vi "PCSMain.set i Attri.vi"(2 "error in (no error)":errorcluster, 3 "systemID":string) -> (0 "error out":errorcluster, 1 "i attribute":T1)   [LabVIEW 2014, in "PCSMain.lvlib"]
uses:
  PCSMain.lvlib
  PCSMain.i attribute.ctl
  PH_Common/PH_Common.lvlib
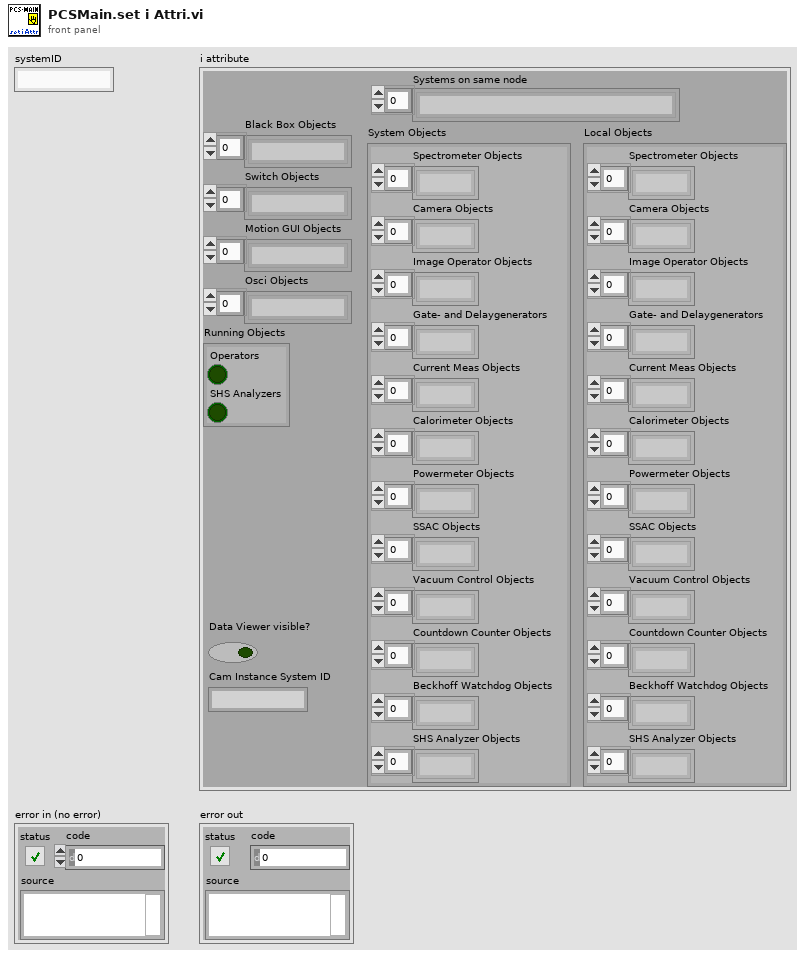
[diagram p1: front panel]
types:
  T1 = typedef "PCSMain.lvlib/PCSMain.i attribute.ctl" = cluster{"System Objects":cluster{"Spectrometer Objects":string[], "Camera Objects":string[], "Image Operator Objects":string[], "Gate- and Delaygenerators":string[], "Current Meas Objects":string[], "Calorimeter Objects":string[], "Powermeter Objects":string[], "SSAC Objects":string[], "Vacuum Control Objects":string[], "Countdown Counter Objects":string[], "Beckhoff Watchdog Objects":string[], "SHS Analyzer Objects":string[]}, "Local Objects":cluster{"Spectrometer Objects":string[], "Camera Objects":string[], "Image Operator Objects":string[], "Gate- and Delaygenerators":string[], "Current Meas Objects":string[], "Calorimeter Objects":string[], "Powermeter Objects":string[], "SSAC Objects":string[], "Vacuum Control Objects":string[], "Countdown Counter Objects":string[], "Beckhoff Watchdog Objects":string[], "SHS Analyzer Objects":string[]}, "Systems on same node":string[], "Data Viewer visible?":bool, "Running Objects":cluster{"Operators":bool, "SHS Analyzers":bool}, "Cam Instance System ID":string, "Black Box Objects":string[], "Switch Objects":string[], "Motion GUI Objects":string[], "Osci Objects":string[]}
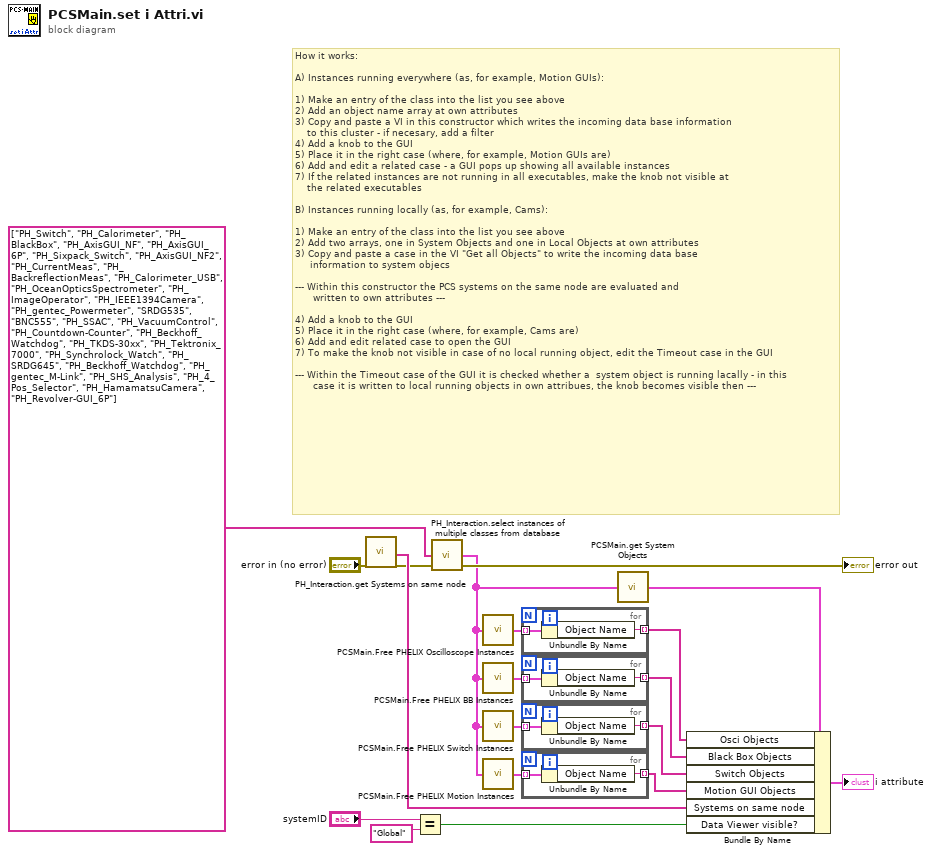
[diagram p0: block diagram]
diagram:
  # "How it works:\n\nA) Instances running everywhere (as, for example, Motion GUIs):\n\n1) Make an entry of the class into the list you see above\n2) Add an object name array at own attributes\n3) Copy and paste a VI in this constructor which writes the incoming data base information \n    to this cluster - if necesary, add a filter\n4) Add a knob to the GUI\n5) Place it in the right case (where, for example, Motion GUIs are)\n6) Add and edit a related case - a GUI pops up showing all available instances\n7) If the related instances are not running in all executables, make the knob not visible at \n    the related executables\n\nB) Instances running locally (as, for example, Cams):\n\n1) Make an entry of the class into the list you see above\n2) Add two arrays, one in System Objects and one in Local Objects at own attributes\n3) Copy and paste a case in the VI \"Get all Objects\" to write the incoming data base \n     information to system objecs\n\n--- Within this constructor the PCS systems on the same node are evaluated and \n      written to own attributes ---\n\n4) Add a knob to the GUI\n5) Place it in the right case (where, for example, Cams are)\n6) Add and edit related case to open the GUI\n7) To make the knob not visible in case of no local running object, edit the Timeout case in the GUI\n\n--- Within the Timeout case of the GUI it is checked whether a  system object is running lacally - in this \n      case it is written to local running objects in own attribues, the knob becomes visible then ---"
  n1 = call "PH_Interaction.get Systems on same node.vi"("error in"="error in (no error)") -> ("List of systems on the same node"=w19:string[], "error out"=w13:errorcluster)  [unwired: 17 in]
  n2 = Equal?(x="systemID", y="Global") -> (x = y?=w17:bool)
  n3 = call "PH_Interaction.select instances of multiple classes from database.vi"("error in (no error)"=w13, "Classes Input"=string[] ["PH_Switch", "PH_Calorimeter", "PH_BlackBox", "PH_AxisGUI_NF", "PH_AxisGUI_6P", "PH_Sixpack_Switch", "PH_AxisGUI_NF2", "PH_CurrentMeas", "PH_BackreflectionMeas", "PH_Calorimeter_USB", "PH_OceanOpticsSpectrometer", "PH_ImageOperator", "PH_IEEE1394Camera", "PH_gentec_Powermeter", "SRDG535", "BNC555", "PH_SSAC", "PH_VacuumControl", "PH_Countdown-Counter", "PH_Beckhoff_Watchdog", "PH_TKDS-30xx", "PH_Tektronix_7000", "PH_Synchrolock_Watch", "PH_SRDG645", "PH_Beckhoff_Watchdog", "PH_gentec_M-Link", "PH_SHS_Analysis", "PH_4_Pos_Selector", "PH_HamamatsuCamera", "PH_Revolver-GUI_6P"]) -> ("error out"=→"error out":errorcluster, "Query Result"=w2:cluster{"Object Name":string, "Class":string}[])  [unwired: 2 in]
  n4 = call "PCSMain.Free PHELIX Oscilloscope Instances.vi"("DB Entries"=w2) -> ("Free Oscilloscope Instances"=w4:cluster{"Object Name":string, "Class":string}[])
  n5 = call "PCSMain.Free PHELIX BB Instances.vi"("DB Entries"=w2) -> ("Free BB Instances"=w6:cluster{"Object Name":string, "Class":string}[])
  n6 = call "PCSMain.Free PHELIX Switch Instances.vi"("DB Entries"=w2) -> ("Free Switch GUI elements"=w8:cluster{"Object Name":string, "Class":string}[])
  n7 = call "PCSMain.Free PHELIX Motion Instances.vi"("DB Entries"=w2) -> ("Free Motion GUI elements"=w10:cluster{"Object Name":string, "Class":string}[])
  n8 = for {
    tunnel: w4 -> [w21] mode=indexing
    tunnel: [w20] -> w3 mode=indexing
    n9 = Unbundle By Name(w21) -> ("Object Name"=w20:string)
  }
  n10 = for {
    tunnel: w6 -> [w23] mode=indexing
    tunnel: [w22] -> w5 mode=indexing
    n11 = Unbundle By Name(w23) -> ("Object Name"=w22:string)
  }
  n12 = for {
    tunnel: w8 -> [w25] mode=indexing
    tunnel: [w24] -> w7 mode=indexing
    n13 = Unbundle By Name(w25) -> ("Object Name"=w24:string)
  }
  n14 = for {
    tunnel: w10 -> [w27] mode=indexing
    tunnel: [w26] -> w9 mode=indexing
    n15 = Unbundle By Name(w27) -> ("Object Name"=w26:string)
  }
  n16 = call "PCSMain.get System Objects.vi"("DB Entries"=w2) -> ("Many i attributes"=w1:T1)
  n17 = Bundle By Name(cluster=w1, "Osci Objects"=w3, "Black Box Objects"=w5, "Switch Objects"=w7, "Motion GUI Objects"=w9, "Systems on same node"=w19, "Data Viewer visible?"=w17) -> (→"i attribute":T1)
